vi "Laser_power_control_slider_calculator.vi"(11 "Laser 488 nm power":dbl(slide) min=0.0 max=5.0 scale=0.0..5.0) -> (2 "Amplitude":dbl, 3 "Offset":dbl)   [LabVIEW 2020]
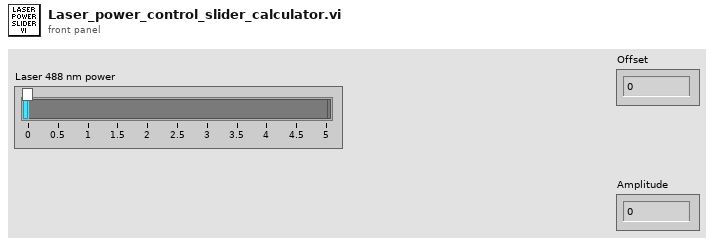
[diagram p1: front panel]
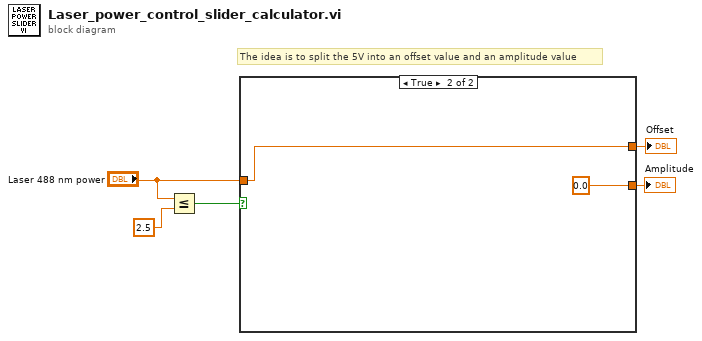
[diagram p0: block diagram]
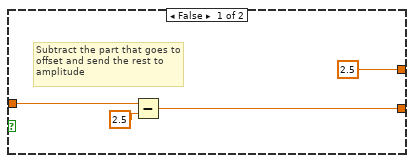
[diagram p2: hidden frame]
diagram:
  # "The idea is to split the 5V into an offset value and an amplitude value"
  n1 = Less Or Equal?(x="Laser 488 nm power", y=2.5) -> (x <= y?=w3:bool)
  n2 = case shown="True" w3 {
    tunnel: "Laser 488 nm power" -> [w8 w11]
    tunnel: [2.5 ("Laser 488 nm power") w11] -> w2
    tunnel: [w6 0.0] -> w1
    frame False {
      # "Subtract the part that goes to offset and send the rest to amplitude"
      n3 = Subtract(x=w8, y=2.5) -> (x-y=w6:dbl)
    }
    frame True {
    }
  }
  "Offset" <- w2
  "Amplitude" <- w1
